vi "PointInRect.vi"(8 "错误输入":errorcluster, 10 "point":cluster{"x":dbl, "y":dbl} caption="点" {"y" format="%.2f"; "x" format="%.2f"}, 11 "rect":T1 caption="矩形") -> (0 "错误输出":errorcluster, 2 "pt in rect":bool caption="矩形中的点")   [LabVIEW 2012, in "Picture Box Tools.lvlib" / "Rect Tools.lvlib"]
uses:
  Rect Tools.lvlib
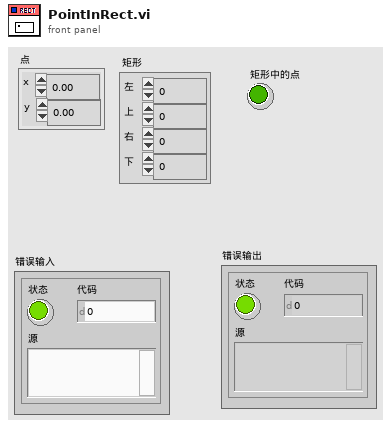
[diagram p1: front panel]
types:
  T1 = cluster{"left":i16, "top":i16, "right":i16, "bottom":i16}
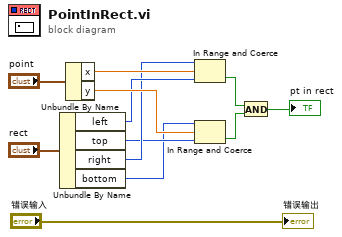
[diagram p0: block diagram]
diagram:
  n1 = Unbundle By Name("rect") -> ("left"=w8:i16, "top"=w6:i16, "right"=w7:i16, "bottom"=w5:i16)
  n2 = Unbundle By Name("point") -> ("x"=w10:dbl, "y"=w9:dbl)
  n3 = In Range and Coerce(upper limit=w7, x=w10, lower limit=w8) -> (In Range?=w4:bool)  [unwired: 1 out]
  n4 = In Range and Coerce(upper limit=w5, x=w9, lower limit=w6) -> (In Range?=w3:bool)  [unwired: 1 out]
  n5 = And(x=w4, y=w3) -> (x .and. y?=→"pt in rect":bool)
  "错误输出" <- "错误输入"
